vi "SCE_parse_VIC_reg_D018.vi"(11 "$D000 - $D03F":u8[](array[numeric]) format="%.0x") -> (3 "VIC-II D018":T1 {"video ram addr" format="%.0x"; "charset addr" format="%.0x"})   [LabVIEW 2018]
uses:
  SCE_VIC-II_reg_D018.ctl
panel:
  # "11"
  # "16"
  # "18"
  # "20"
  # "21"
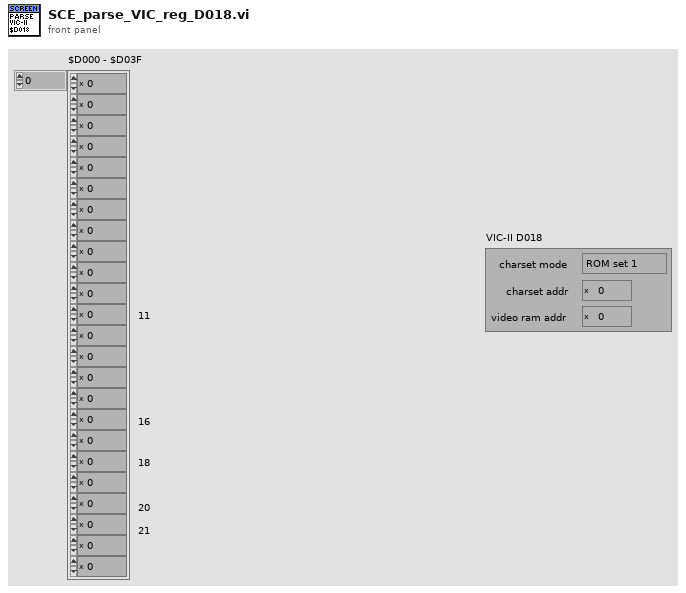
[diagram p1: front panel]
types:
  T1 = typedef "SCE_VIC-II_reg_D018.ctl" = cluster{"charset mode":enum16{"ROM set 1", "ROM set 2", "RAM"}, "charset addr":u16, "video ram addr":u16}
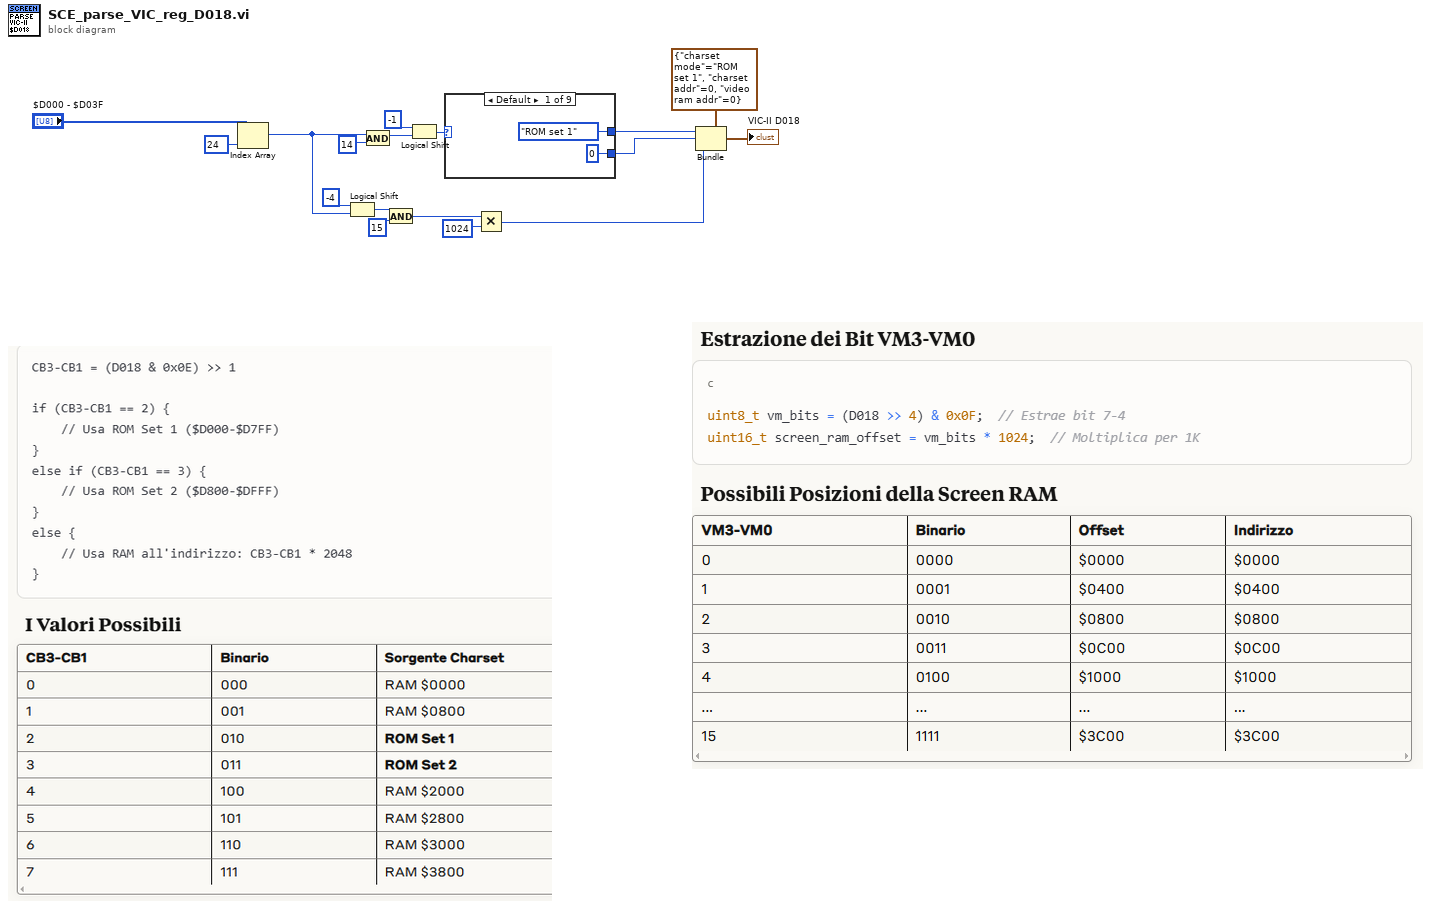
[diagram p0: block diagram]
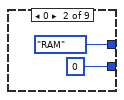
[diagram p2: hidden frame]
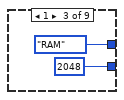
[diagram p3: hidden frame]
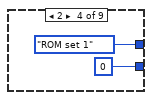
[diagram p4: hidden frame]
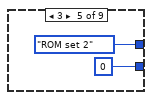
[diagram p5: hidden frame]
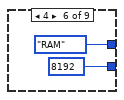
[diagram p6: hidden frame]
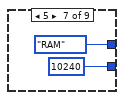
[diagram p7: hidden frame]
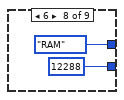
[diagram p8: hidden frame]
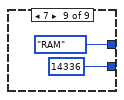
[diagram p9: hidden frame]
diagram:
  n1 = Index Array(array="$D000 - $D03F", index=24) -> (element=w3:u8)
  n2 = Logical Shift(y=-4 ("x"), x=w3) -> (x << y=w2:u8)
  n3 = And(x=w3, y=u8 14 ("index")) -> (x .and. y?=w5:u8)
  n4 = And(x=w2, y=u8 15 ("index")) -> (x .and. y?=w9:u8)
  n5 = Logical Shift(y=-1 ("x"), x=w5) -> (x << y=w6:u8)
  n6 = case shown="Default" w6 {
    tunnel: [enum16{"ROM set 1", "ROM set 2", "RAM"}."ROM set 1" ("charset mode") enum16{"ROM set 1", "ROM set 2", "RAM"}."RAM" ("charset mode") enum16{"ROM set 1", "ROM set 2", "RAM"}."RAM" ("charset mode") enum16{"ROM set 1", "ROM set 2", "RAM"}."ROM set 1" ("charset mode") enum16{"ROM set 1", "ROM set 2", "RAM"}."ROM set 2" ("charset mode") enum16{"ROM set 1", "ROM set 2", "RAM"}."RAM" ("charset mode") enum16{"ROM set 1", "ROM set 2", "RAM"}."RAM" ("charset mode") enum16{"ROM set 1", "ROM set 2", "RAM"}."RAM" ("charset mode") enum16{"ROM set 1", "ROM set 2", "RAM"}."RAM" ("charset mode")] -> w13
    tunnel: [u16 0 ("charset addr") u16 0 ("charset addr") u16 2048 ("charset addr") u16 0 ("charset addr") u16 0 ("charset addr") u16 8192 ("charset addr") u16 10240 ("charset addr") u16 12288 ("charset addr") u16 14336 ("charset addr")] -> w11
    frame Default {
    }
    frame 0 {
    }
    frame 1 {
    }
    frame 2 {
    }
    frame 3 {
    }
    frame 4 {
    }
    frame 5 {
    }
    frame 6 {
    }
    frame 7 {
    }
  }
  n7 = Multiply(x=w9, y=u16 1024 ("charset addr")) -> (x*y=w7:u16)
  n8 = Bundle(cluster=T1 {"charset mode"=enum."ROM set 1", "charset addr"=0, "video ram addr"=0} ("VIC-II D018"), "charset mode"=w13, "charset addr"=w11, "video ram addr"=w7) -> (→"VIC-II D018":T1)
